vi "Ellipse Contour Points.vi"(0 "A":dbl(slide)=10.0 scale=0.0..100.0, 2 "rotation":dbl(slide) scale=0.0..180.0, 5 "B":dbl(slide)=10.0 scale=0.0..100.0, 7 "x-Shift":dbl(slide) scale=-50.0..50.0, 9 "y-shift":dbl(slide) scale=-50.0..50.0, 11 "error in":errorcluster) -> (4 "Contour Array Points":dbl[][](array[numeric]), 15 "error out":errorcluster)   [LabVIEW 2014]
doc: "Calculates contour points of an ellipse\n\nx- and y-Shift represent the center of the ellipse\nA and B define the width and height\nrotation is the rotation angle"
panel:
  out "XY Graph":cluster{dbl[], dbl[]}(graph)
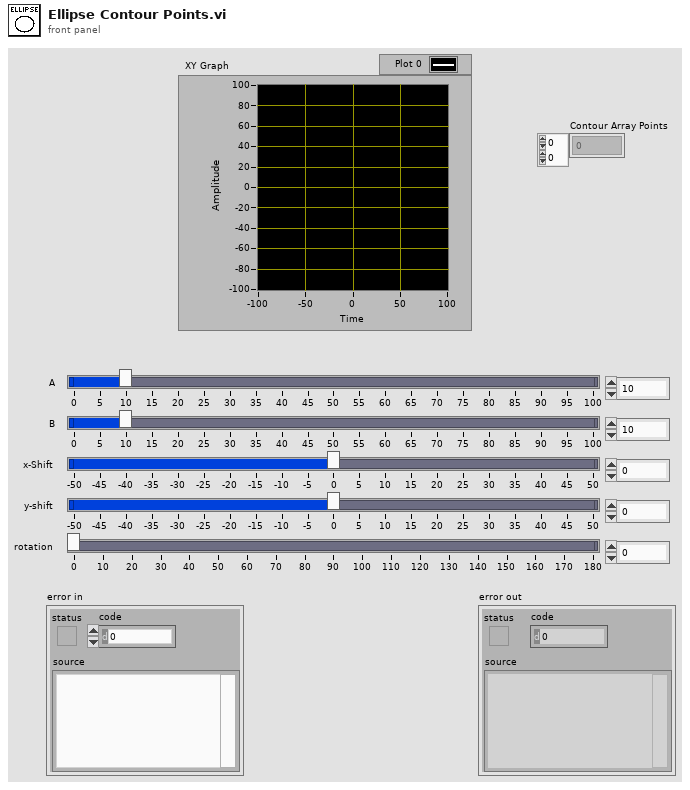
[diagram p1: front panel]
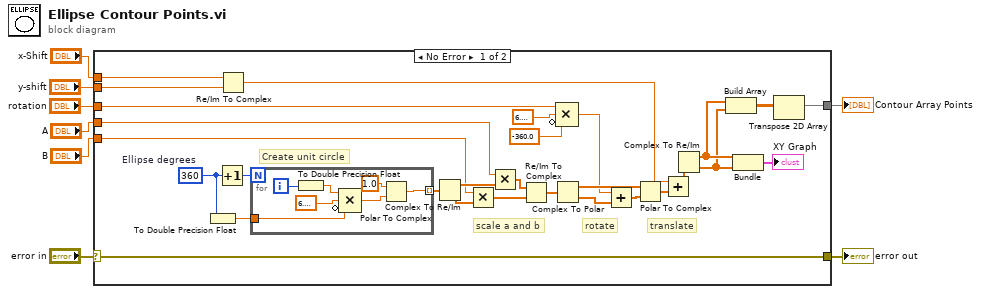
[diagram p0: block diagram]
diagram:
  n1 = case shown="No Error" "error in" {
    selector: "error in" -> [w13 w45]
    tunnel: "rotation" -> [w23 _]
    tunnel: "A" -> [w19 _]
    tunnel: "B" -> [w18 _]
    tunnel: "x-Shift" -> [w17 _]
    tunnel: "y-shift" -> [w16 _]
    tunnel: [w13 w45] -> w2
    tunnel: [w9 _] -> w1
    frame No Error {
      w35 = 360  # Ellipse degrees
      # "translate"
      # "rotate"
      # "scale a and b"
      # "Create unit circle"
      # "http://forums.ni.com/t5/LabVIEW/build-an-ellipse-and-plot-it/m-p/262058#M140604"
      n2 = To Double Precision Float(number=w35) -> (double precision float=w37:dbl)
      n3 = Increment(x=w35) -> (x+1=w15:i32)
      n4 = Re/Im To Complex(1:w16, 2:w17) -> (0:w24:cdb)
      n5 = for {
        N: w15 -> [_]
        tunnel: w37 -> [w38]
        tunnel: [w42] -> w34 mode=indexing
        i -> [w43]
        n6 = To Double Precision Float(number=w43) -> (double precision float=w40:dbl)
        n7 = Compound Arithmetic op=MULTIPLY(w40, 6.283185307179586, invert w38) -> (w39:dbl)
        n8 = Polar To Complex(1:w39, 2:1.0 ("r")) -> (0:w42:cdb)
      }
      n9 = Complex To Re/Im(x + iy=w34) -> (x=w33:dbl[], y=w36:dbl[])
      n10 = Multiply(x=w18, y=w36) -> (x*y=w31:dbl[])
      n11 = Multiply(x=w19, y=w33) -> (x*y=w32:dbl[])
      n12 = Re/Im To Complex(1:w31, 2:w32) -> (0:w30:cdb[])
      n13 = Complex To Polar(r * e^(i*theta)=w30) -> (r=w28:dbl[], theta=w29:dbl[])
      n14 = Compound Arithmetic op=MULTIPLY(w23, 6.283185307179586, invert -360.0 ("y")) -> (w20:dbl)
      n15 = Add(x=w20, y=w29) -> (x+y=w27:dbl[])
      n16 = Polar To Complex(1:w27, 2:w28) -> (0:w26:cdb[])
      n17 = Add(x=w24, y=w26) -> (x+y=w25:cdb[])
      n18 = Complex To Re/Im(x + iy=w25) -> (x=w12:dbl[], y=w11:dbl[])
      n19 = Build Array(w12, w11) -> (w10:dbl[][])
      n20 = Bundle(w12, w11) -> (→"XY Graph":cluster{dbl[], dbl[]})  [unwired: 1 in]
      n21 = Transpose 2D Array(2D array=w10) -> (transposed array=w9:dbl[][])
    }
    frame Error {
    }
  }
  "error out" <- w2
  "Contour Array Points" <- w1
